vi "test Encode and Decode (BCD, unsigned).vi"(8 "error in (no error)":errorcluster, 11 "TestCase in":refnum<class "Encoding and Decoding.lvclass">) -> (0 "error out":errorcluster, 3 "TestCase out":refnum<class "Encoding and Decoding.lvclass">)   [LabVIEW 2020, in "Encoding and Decoding.lvclass"]
uses:
  Encoding and Decoding.lvclass
  Protocol/Implementations/ARINC429/Parameter Definition.ctl
  Encoding and Decoding/Encoding.ctl
  Protocol/Implementations/ARINC429/ARINC429-32bit/32-bit Word.lvclass/32-bit Word.ctl
  4413749d-09be-4b2c-9fd8-42957a21c6ba.vi
  Shared/Encode Parameter and Update Word (32-bit).vi/1445f95d-237d-4fc6-96b9-8992d347f513.vi
  Shared/Encode Parameter and Update Word (32-bit).vi/6b8853f0-8e5d-49e3-9391-4d3f8e5314b0.vi
  Shared/Encode Parameter and Update Word (32-bit).vi/2babc4f4-546e-4d35-846d-a4a1fbac0249.vi
  4413749d-09be-4b2c-9fd8-42957a21c6ba.vi/f69091ce-4ebb-4c6c-86d4-95f2f98c0ab9.vi
  4413749d-09be-4b2c-9fd8-42957a21c6ba.vi/bd4d0fb3-691f-452d-8155-40a0d56859ad.vi
  Shared/Encode Parameter and Update Word (32-bit).vi/1445f95d-237d-4fc6-96b9-8992d347f513.vi/22abf0d2-70bd-4b51-a478-b97a2704f7df.vi
  Shared/Encode Parameter and Update Word (32-bit).vi/1445f95d-237d-4fc6-96b9-8992d347f513.vi/c253b733-33bf-43c6-b07a-ea22f5c7a6f3.vi
  Shared/Encode Parameter and Update Word (32-bit).vi/1445f95d-237d-4fc6-96b9-8992d347f513.vi/9377bb8f-44b5-4a8f-87f1-966fd5a9edcc.vi
  Shared/Encode Parameter and Update Word (32-bit).vi/6b8853f0-8e5d-49e3-9391-4d3f8e5314b0.vi/a54b505c-1216-4ef4-8378-3ceda9d188df.vi
  Shared/Encode Parameter and Update Word (32-bit).vi/6b8853f0-8e5d-49e3-9391-4d3f8e5314b0.vi/136dcdcb-2dd3-4a4d-a796-a8f7a3f8e1ac.vi
  4413749d-09be-4b2c-9fd8-42957a21c6ba.vi/f69091ce-4ebb-4c6c-86d4-95f2f98c0ab9.vi/16a2565b-3c16-407b-a626-9da2a3da432e.vi
  4413749d-09be-4b2c-9fd8-42957a21c6ba.vi/bd4d0fb3-691f-452d-8155-40a0d56859ad.vi/0a001d06-2809-4638-8d0b-e017d2157007.vi
  Encoding and Decoding/BCD Decode Integer.vi
  Shared/Encode Parameter and Update Word (32-bit).vi/1445f95d-237d-4fc6-96b9-8992d347f513.vi/22abf0d2-70bd-4b51-a478-b97a2704f7df.vi/9d450a76-0fc9-4555-8e71-4c202274969f.vi
  Shared/Encode Parameter and Update Word (32-bit).vi/1445f95d-237d-4fc6-96b9-8992d347f513.vi/c253b733-33bf-43c6-b07a-ea22f5c7a6f3.vi/9d450a76-0fc9-4555-8e71-4c202274969f.vi
  Shared/Encode Parameter and Update Word (32-bit).vi/6b8853f0-8e5d-49e3-9391-4d3f8e5314b0.vi/a54b505c-1216-4ef4-8378-3ceda9d188df.vi/a7fcce85-1f75-4572-aeaa-ddfd463a7c5f.vi
  Encoding and Decoding/BCD Decode Integer.vi/9a65bfc0-0d77-4ef3-ab58-63df1e1caa90.vi
  Protocol/Implementations/ARINC429/ARINC429-32bit/32-bit Word.lvclass
  <vilib>/addons/_JKI Toolkits/VI Tester/TestCase.llb/TestCase.lvclass
  Encoding and Decoding/Encoding and Decoding.lvlib
  Protocol/Implementations/ARINC429/ARINC 429.lvclass
  C:/Program Files (x86)/National Instruments/LabVIEW 2020/vi.lib/addons/_JKI Toolkits/VI Tester/TestCase.llb/TestCase.lvclass
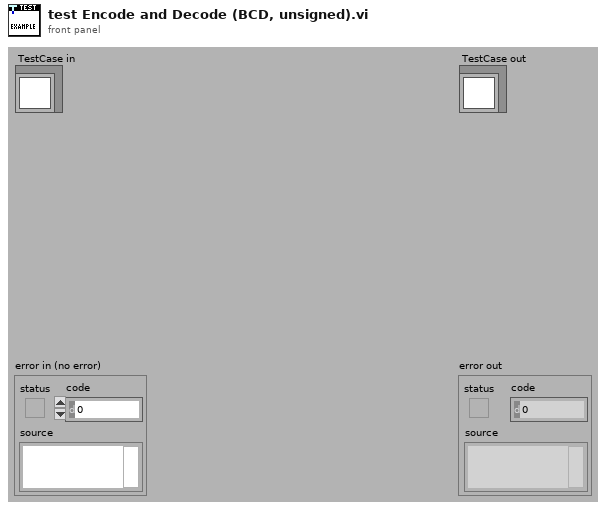
[diagram p1: front panel]
types:
  T1 = typedef "ARINC 429.lvclass/Parameter Definition.ctl" = cluster{"start index":i32, "size":i32, "encoding":T2, "signed":bool, "scale multiplier":dbl, "scale offset":dbl}
  T2 = typedef "Encoding and Decoding.lvlib/Encoding.ctl" = enum16{"BNR", "BCD", "Discrete"}
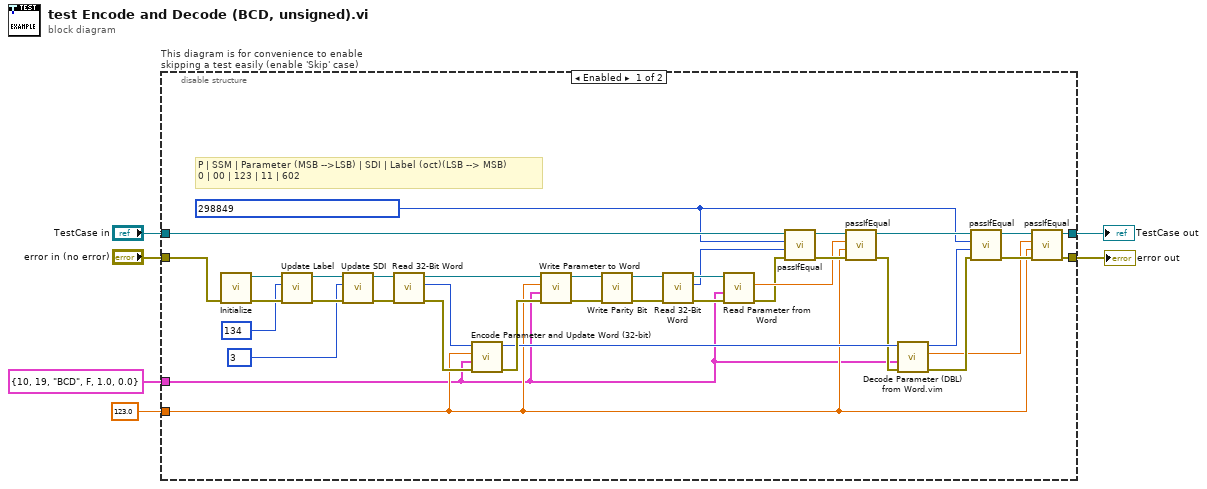
[diagram p0: block diagram]
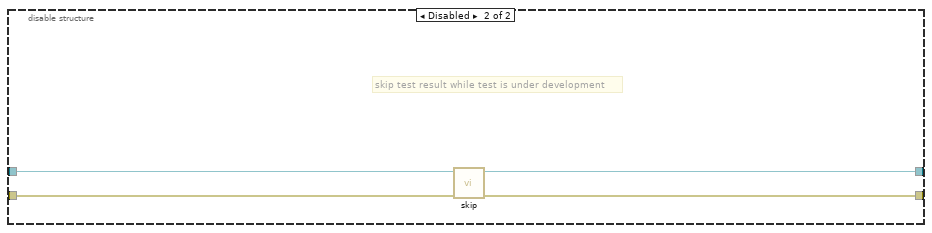
[diagram p2: hidden frame]
diagram:
  n1 = disable-structure "This diagram is for convenience to enable skipping a test easily (enable 'Skip' case)" shown="Enabled" {
    disable-tunnel: "TestCase in" -> [w27 w48]
    disable-tunnel: [w16 w46] -> w3
    disable-tunnel: [w15 w47] -> w5
    disable-tunnel: "error in (no error)" -> [w26 w45]
    disable-tunnel: T1 {"start index"=10, "size"=19, "encoding"=enum."BCD", "signed"=FALSE, "scale multiplier"=1.0, "scale offset"=0.0} ("parameter definition") -> [w7 _]
    disable-tunnel: 123.0 ("parameter value") -> [w10 _]
    frame Enabled {
      w8 = u32 298849 ("SDI value 2")
      # "P | SSM | Parameter (MSB -->LSB) | SDI | Label (oct)(LSB --> MSB)\n0 | 00 | 123 | 11 | 602"
      n2 = call "Initialize.vi"("error in"=w26) -> ("error out"=w38:errorcluster, "ARINC 429 (32-bit word)"=w33:refnum<class "32-bit Word.lvclass">)  [unwired: 9 in]
      n3 = call-dynamic "Update Label.vi"("error in"=w38, "label value"=u8 134 ("label value 2"), "32-bit word in"=w33) -> ("error out"=w39:errorcluster, "32-bit word out"=w36:refnum<class "32-bit Word.lvclass">)  [unwired: 7 in]
      n4 = call-dynamic "Update SDI.vi"("error in"=w39, "SDI value"=u8 3 ("SDI value 2"), "32-bit Word in"=w36) -> ("error out"=w24:errorcluster, "32-bit Word out"=w25:refnum<class "32-bit Word.lvclass">)  [unwired: 7 in]
      n5 = call "Read 32-Bit Word.vi"("error in (no error)"=w24, "32-bit Word in"=w25) -> ("error out"=w21:errorcluster, "32-bit word"=w22:u32, "32-bit Word out"=w23:refnum<class "32-bit Word.lvclass">)  [unwired: 7 in]
      n6 = call "Encode Parameter and Update Word (32-bit).vi"("error in"=w21, "parameter definition"=w7, "parameter value"=w10, "word in"=w22) -> ("error out"=w20:errorcluster, "word out"=w19:u32)  [unwired: 6 in]
      n7 = call-dynamic "Write Parameter to Word.vi"("error in"=w20, "parameter definition"=w7, "data"=w10, "32-bit Word in"=w23) -> ("error out"=w41:errorcluster, "32-bit Word out"=w42:refnum<class "32-bit Word.lvclass">)  [unwired: 6 in]
      n8 = call-dynamic "Write Parity Bit.vi"("error in"=w41, "32-bit word in"=w42) -> ("error out"=w40:errorcluster, "32-bit word out"=w37:refnum<class "32-bit Word.lvclass">)  [unwired: 8 in]
      n9 = call "Read 32-Bit Word.vi"("error in (no error)"=w40, "32-bit Word in"=w37) -> ("error out"=w44:errorcluster, "32-bit word"=w29:u32, "32-bit Word out"=w43:refnum<class "32-bit Word.lvclass">)  [unwired: 7 in]
      n10 = call-dynamic "Read Parameter from Word.vi"("error in"=w44, "parameter definition"=w7, "32-bit Word in"=w43) -> ("error out"=w28:errorcluster, "parameter value"=w30:dbl)  [unwired: 6 in, 1 out]
      n11 = call-dynamic "passIfEqual.vi"("error in (no error)"=w28, "y"=w29, "x"=w8, "TestCase in"=w27) -> ("error out"=w31:errorcluster, "TestCase out"=w32:refnum<class "Encoding and Decoding.lvclass">)  [unwired: 6 in]
      n12 = call-dynamic "passIfEqual.vi"("error in (no error)"=w31, "y"=w10, "x"=w30, "TestCase in"=w32) -> ("error out"=w13:errorcluster, "TestCase out"=w14:refnum<class "Encoding and Decoding.lvclass">)  [unwired: 6 in]
      n13 = call "Decode Parameter (DBL) from Word.vim"("error in"=w13, "parameter definition"=w7, "32-bit word in"=w19) -> ("error out"=w12:errorcluster, "parameter value"=w11:dbl, "32-bit word out"=w9:u32)  [unwired: 6 in]
      n14 = call-dynamic "passIfEqual.vi"("error in (no error)"=w12, "y"=w9, "x"=w8, "TestCase in"=w14) -> ("error out"=w18:errorcluster, "TestCase out"=w17:refnum<class "Encoding and Decoding.lvclass">)  [unwired: 6 in]
      n15 = call-dynamic "passIfEqual.vi"("error in (no error)"=w18, "y"=w10, "x"=w11, "TestCase in"=w17) -> ("error out"=w15:errorcluster, "TestCase out"=w16:refnum<class "Encoding and Decoding.lvclass">)  [unwired: 6 in]
    }
    frame Disabled {
      # "skip test result while test is under development"
      n16 = call <vilib>:"skip.vi"("error in (no error)"=w45, "TestCase in"=w48) -> ("error out"=w47:errorcluster, "TestCase out"=w46:refnum<class "Encoding and Decoding.lvclass">)  [unwired: 8 in]
    }
  }
  "error out" <- w5
  "TestCase out" <- w3
